vi "Analyse Double Click.vi"(8 "error in (no error)":errorcluster, 11 "Waveform in":dbl[](graph)) -> (0 "error out":errorcluster, 2 "Number of Valleys":i32, 3 "Valley Indexes":i32[](array[numeric]))   [LabVIEW 2019]
panel:
  out "Amplified Graph":dbl[](graph)
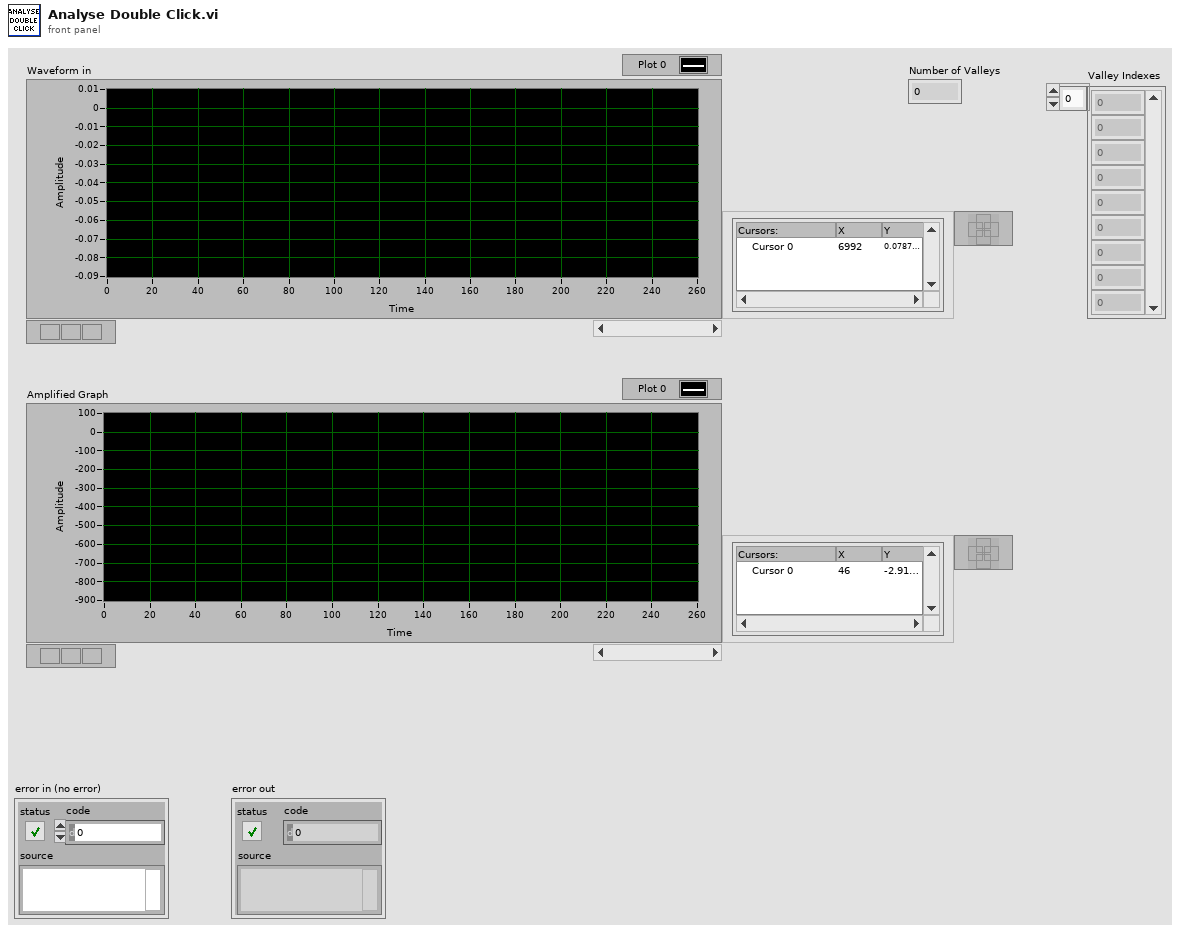
[diagram p1: front panel]
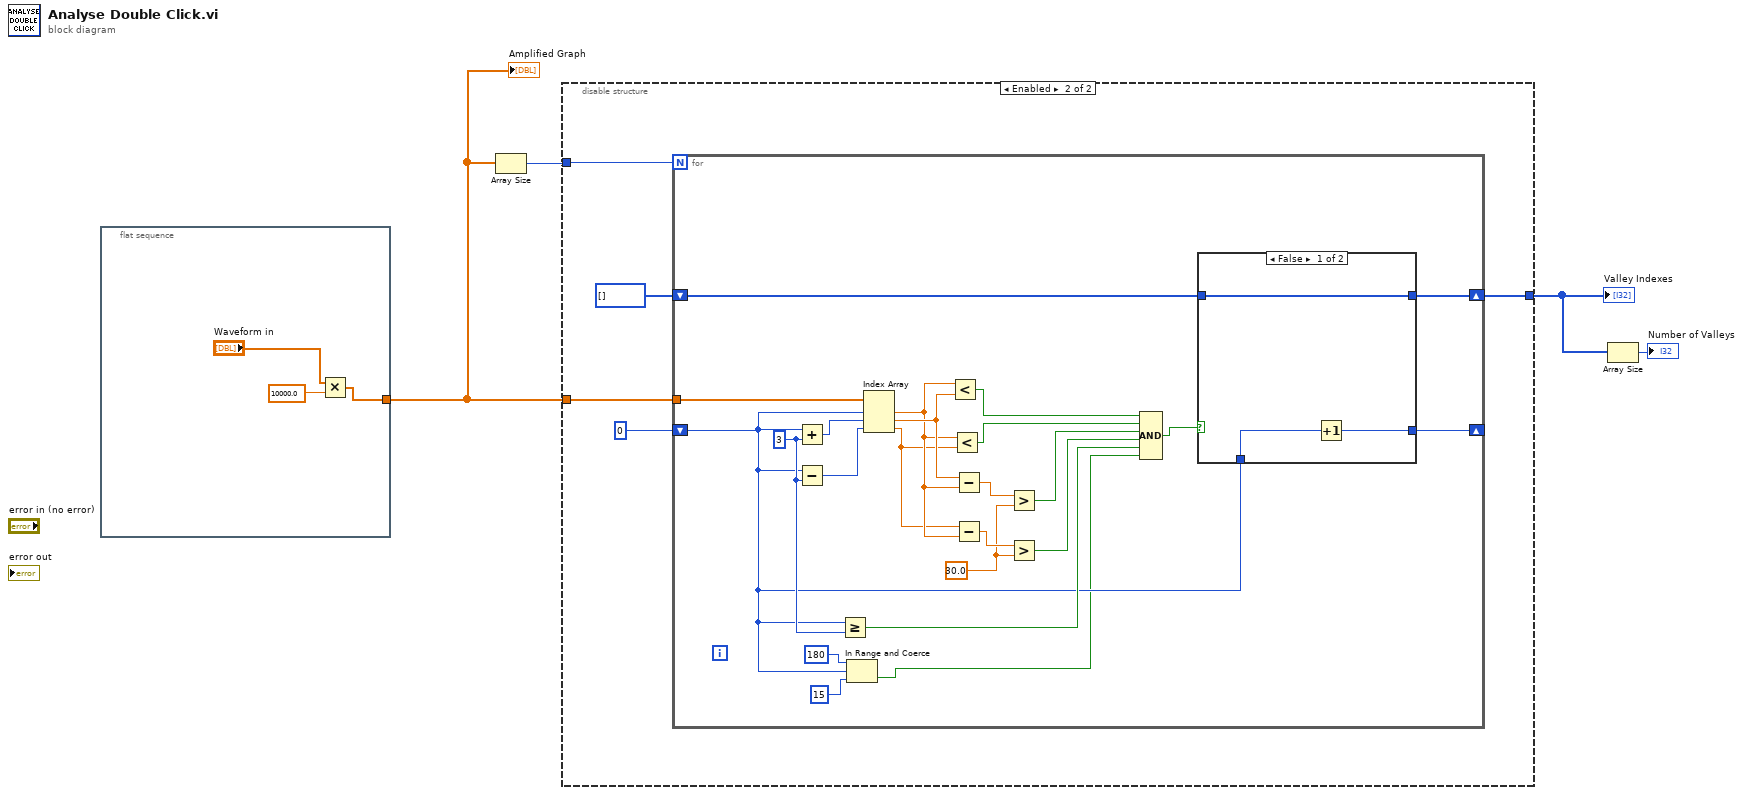
[diagram p0: block diagram]
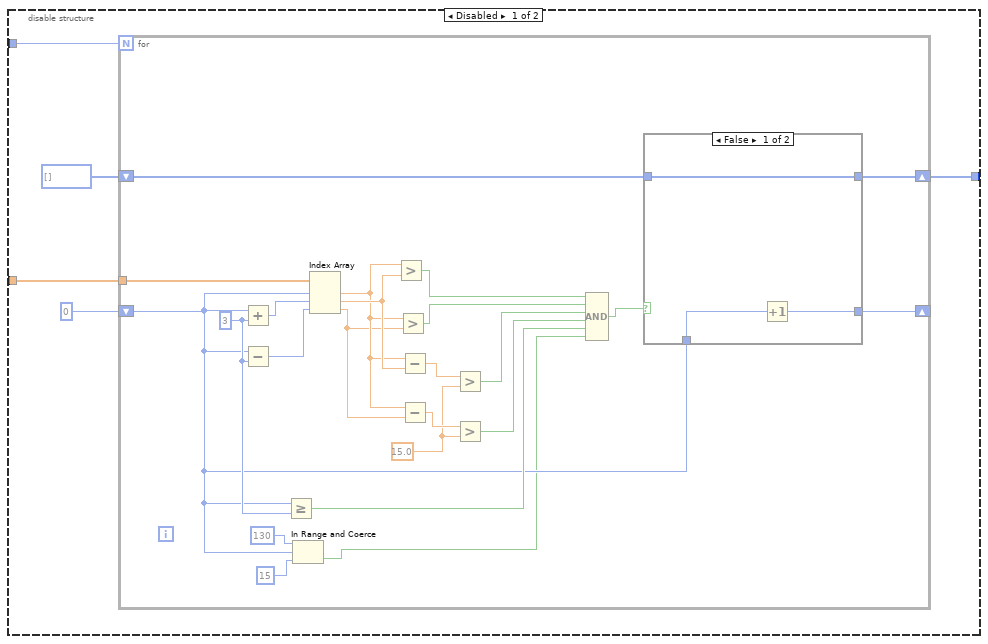
[diagram p2: hidden frame]
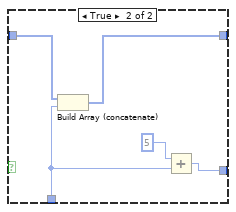
[diagram p3: hidden frame]
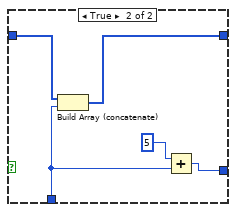
[diagram p4: hidden frame]
diagram:
  n1 = flat-sequence {
    tunnel: [w5] -> w4
    frame #0 {
      n2 = Multiply(x="Waveform in", y=10000.0) -> (x*y=w5:dbl[])
    }
  }
  n3 = Array Size(array=w4) -> (size(s)=w3:i32)
  n4 = disable-structure shown="Enabled" {
    disable-tunnel: w4 -> [w12 w48]
    disable-tunnel: w3 -> [w10 w46]
    disable-tunnel: [w8 w44] -> w2
    frame Disabled {
      n5 = for {
        N: w10 -> [_]
        tunnel: w12 -> [w35]
        shift-right: [w21] -> _
        shift-left: 0 -> [w16]
        shift-right: [w20] -> w8
        shift-left: i32[] [] -> [w19]
        w25 = 15.0 ("y")
        w18 = 3 ("y")
        n6 = Add(x=w16, y=w18) -> (x+y=w33:i32)
        n7 = Subtract(x=w16, y=w18) -> (x-y=w34:i32)
        n8 = Greater Or Equal?(x=w16, y=w18) -> (x >= y?=w17:bool)
        n9 = In Range and Coerce(upper limit=130, x=w16, lower limit=15 ("upper limit")) -> (In Range?=w13:bool)  [unwired: 1 out]
        n10 = Index Array(array=w35, index #1=w16, index #2=w33, index #3=w34) -> (element #1=w29:dbl, element #2=w30:dbl, element #3=w28:dbl)
        n11 = Greater?(x=w29, y=w30) -> (0:w32:bool)
        n12 = Greater?(x=w29, y=w28) -> (0:w31:bool)
        n13 = Subtract(x=w29, y=w30) -> (x-y=w27:dbl)
        n14 = Subtract(x=w29, y=w28) -> (x-y=w26:dbl)
        n15 = Greater?(x=w27, y=w25) -> (0:w24:bool)
        n16 = Greater?(x=w26, y=w25) -> (0:w23:bool)
        n17 = Compound Arithmetic op=AND(w32, w31, w24, w23, w17, w13) -> (w22:bool)
        n18 = case shown="False" w22 {
          tunnel: w16 -> [w38 w42]
          tunnel: [w37 w41] -> w21
          tunnel: [w36 w40] -> w20
          tunnel: w19 -> [w36 w39]
          frame False {
            n19 = Increment(x=w38) -> (x+1=w37:i32)
          }
          frame True {
            n20 = Build Array (concatenate)(w39, w42) -> (w40:i32[])
            n21 = Add(x=5, y=w42) -> (x+y=w41:i32)
          }
        }
      }
    }
    frame Enabled {
      n22 = for {
        N: w46 -> [_]
        tunnel: w48 -> [w71]
        shift-right: [w57] -> _
        shift-left: 0 -> [w52]
        shift-right: [w56] -> w44
        shift-left: i32[] [] -> [w55]
        w61 = 30.0 ("y")
        w54 = 3 ("y")
        n23 = Add(x=w52, y=w54) -> (x+y=w69:i32)
        n24 = Subtract(x=w52, y=w54) -> (x-y=w70:i32)
        n25 = Greater Or Equal?(x=w52, y=w54) -> (x >= y?=w53:bool)
        n26 = In Range and Coerce(upper limit=180, x=w52, lower limit=15 ("upper limit")) -> (In Range?=w49:bool)  [unwired: 1 out]
        n27 = Index Array(array=w71, index #1=w52, index #2=w69, index #3=w70) -> (element #1=w65:dbl, element #2=w66:dbl, element #3=w64:dbl)
        n28 = Less?(x=w65, y=w66) -> (x < y?=w68:bool)
        n29 = Less?(x=w65, y=w64) -> (x < y?=w67:bool)
        n30 = Subtract(x=w66, y=w65) -> (x-y=w63:dbl)
        n31 = Subtract(x=w64, y=w65) -> (x-y=w62:dbl)
        n32 = Greater?(x=w63, y=w61) -> (0:w60:bool)
        n33 = Greater?(x=w62, y=w61) -> (0:w59:bool)
        n34 = Compound Arithmetic op=AND(w68, w67, w60, w59, w53, w49) -> (w58:bool)
        n35 = case shown="False" w58 {
          tunnel: w52 -> [w74 w78]
          tunnel: [w73 w77] -> w57
          tunnel: [w72 w76] -> w56
          tunnel: w55 -> [w72 w75]
          frame False {
            n36 = Increment(x=w74) -> (x+1=w73:i32)
          }
          frame True {
            n37 = Build Array (concatenate)(w75, w78) -> (w76:i32[])
            n38 = Add(x=5, y=w78) -> (x+y=w77:i32)
          }
        }
      }
    }
  }
  "Valley Indexes" <- w2
  n39 = Array Size(array=w2) -> (size(s)=→"Number of Valleys":i32)
  "Amplified Graph" <- w4
